vi "Move.vi"(9 "Team in":refnum<class "Team.lvclass">, 11 "MySquare in":refnum<class "MySquare.lvclass">) -> (1 "Team out":refnum<class "Team.lvclass">, 3 "MySquare out":refnum<class "MySquare.lvclass">)   [LabVIEW 2020, in "DemoTeam.lvlib" / "MySquare.lvclass"]
uses:
  MySquare.lvclass
  SquareBattle/Team/Team.lvclass
  MyTeam/MyTeam.lvclass
  C:/Apps/GIE/Instructions Test/SquareBattle/Team/Team.lvclass
  SquareBattle/Square/Square.lvclass
  C:/Apps/GIE/Instructions Test/SquareBattle/Square/Square.lvclass
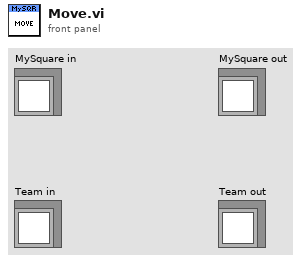
[diagram p1: front panel]
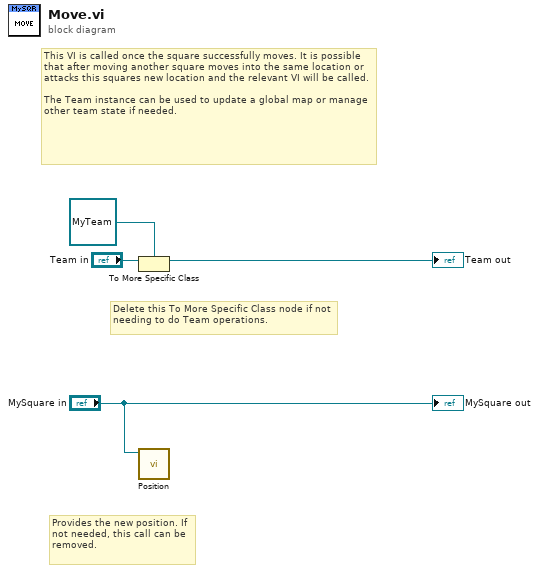
[diagram p0: block diagram]
diagram:
  # "Delete this To More Specific Class node if not needing to do Team operations."
  # "Provides the new position. If not needed, this call can be removed."
  # "This VI is called once the square successfully moves. It is possible that after moving another square moves into the same location or attacks this squares new location and the relevant VI will be called.\n\nThe Team instance can be used to update a global map or manage other team state if needed."
  n1 = To More Specific Class(target class=refnum<class "MyTeam.lvclass"> refnum ("SquareTeam.lvlib:MyTeam.lvclass"), reference="Team in") -> (specific class reference=→"Team out":refnum<class "MyTeam.lvclass">)  [unwired: 1 in, 1 out]
  n2 = call "Position.vi"("Square in"="MySquare in") -> ()  [unwired: 10 in, 1 out]
  "MySquare out" <- "MySquare in"
